vi "Get ctrl Primary Button.vi"(3 "Controls":T1[](array[typedef])) -> (0 "Output":bool[](array[boolean]))   [LabVIEW 2014]
uses:
  TypeDefs/Button Actions.ctl
  TypeDefs/SRE Enum.ctl
  Support Code/Robot Global Data.vi
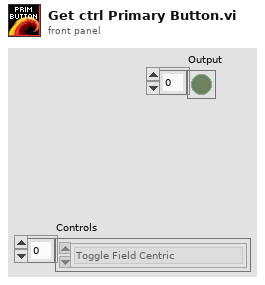
[diagram p1: front panel]
types:
  T1 = typedef "Button Actions.ctl" = enum16{"Gyro Reset", "Toggle Field Centric", "Clear Faults", "Reduce Speed", "Output", "Rotate Left 45", "Rotate Right 45", "Center", "Chute Door", "Strafe Right", "Strafe Left", "Strafe Down", "Strafe Up"}
  T2 = typedef "SRE Enum.ctl" = enum16{"Start", "Run", "End"}
  T3 = enum16{"Trigger Left", "2 Left", "3 Left", "4 Left", "5 Left", "6 Left", "7 Left", "8 Left", "9 Left", "10 Left", "11 Left", "Trigger Right", "2 Right", "3 Right", "4 Right", "5 Right", "6 Right", "7 Right", "8 Right", "9 Right", "10 Right", "11 Right"}[]
  T4 = enum16{"Trigger Left", "2 Left", "3 Left", "4 Left", "5 Left", "6 Left", "7 Left", "8 Left", "9 Left", "10 Left", "11 Left", "Trigger Right", "2 Right", "3 Right", "4 Right", "5 Right", "6 Right", "7 Right", "8 Right", "9 Right", "10 Right", "11 Right"}
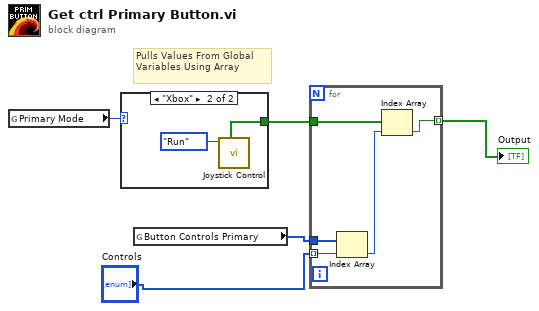
[diagram p0: block diagram]
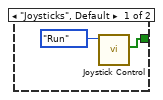
[diagram p2: hidden frame]
diagram:
  # "Pulls Values From Global Variables Using Array"
  n1 = global read "Robot Global Data.vi" "Primary Mode"() -> (w5:enum16{"Joysticks", "Xbox"})
  n2 = case shown="\"Xbox\"" w5 {
    tunnel: [w6 w8] -> w2
    frame "Joysticks", Default {
      n3 = call "Joystick Control.vi"("Enum"=SRE_Enum."Run") -> ("Button Output PJ"=w6:bool[])  [unwired: 3 in, 5 out]
    }
    frame "Xbox" {
      n4 = call "Joystick Control.vi"("Enum"=SRE_Enum."Run") -> ("Buttons Output PX"=w8:bool[])  [unwired: 3 in, 5 out]
    }
  }
  n5 = global read "Robot Global Data.vi" "Button Controls Primary"() -> (w4:T3)
  n6 = for {
    tunnel: "Controls" -> [w14] mode=indexing
    tunnel: w4 -> [w13]
    tunnel: w2 -> [w11]
    tunnel: [w10] -> w1 mode=indexing
    n7 = Index Array(array=w13, index=w14) -> (element=w12:T4)
    n8 = Index Array(array=w11, index=w12) -> (element=w10:bool)
  }
  "Output" <- w1
